vi "SetIMAvg.vi"(6 "Legacy (f)?":bool, 8 "error in (no error)":errorcluster, 10 "SetIMAvg":T1 items=["None", "Minimum", "Normal", "High", "Maximum"]) -> (0 "error out":errorcluster)   [LabVIEW 2011]
uses:
  HW Averaging.ctl
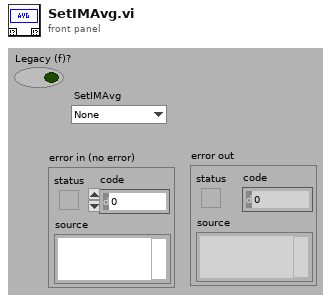
[diagram p1: front panel]
types:
  T1 = typedef "HW Averaging.ctl" = u16
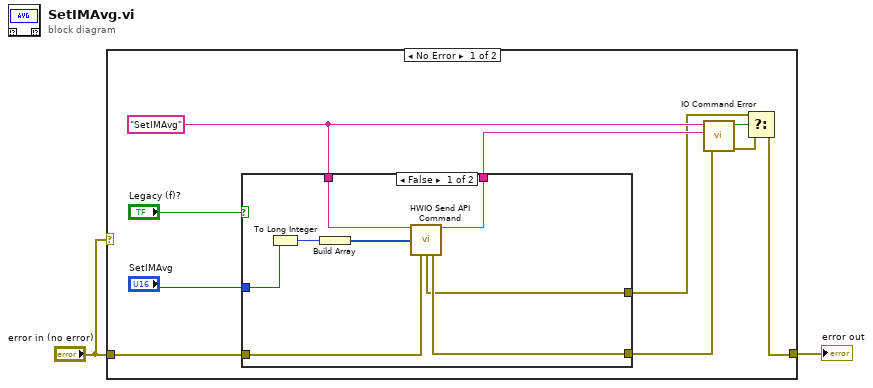
[diagram p0: block diagram]
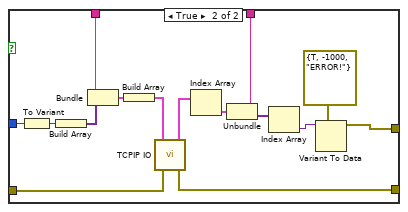
[diagram p2: hidden frame]
diagram:
  n1 = case shown="No Error" "error in (no error)" {
    tunnel: "error in (no error)" -> [w11 w36]
    tunnel: [w6 w36] -> w2
    frame No Error {
      w9 = "SetIMAvg"
      n2 = case shown="False" "Legacy (f)?" {
        tunnel: "SetIMAvg" -> [w16 w33]
        tunnel: w11 -> [w20 w32]
        tunnel: [w19 w30] -> w10
        tunnel: w9 -> [w17 w29]
        tunnel: [w18 w26] -> w8
        tunnel: [w13 w21] -> w4
        frame False {
          n3 = To Long Integer(number=w16) -> (32bit integer=w15:i32)
          n4 = Build Array(w15) -> (w14:i32[])
          n5 = call "HWIO Send API Command.vi"("Action"=w17, "Integer"=w14, "error in (no error)"=w20) -> ("Action out"=w18:string, "HWError"=w13:errorcluster, "error out"=w19:errorcluster)  [unwired: 5 in, 5 out]
        }
        frame True {
          n6 = To Variant(anything=w33) -> (Variant=w35:variant)
          n7 = Build Array(w35) -> (w34:variant[])
          n8 = Bundle(w29, w34) -> (w31:cluster{string, variant[]})  [unwired: 1 out]
          n9 = Build Array(w31) -> (w28:cluster{string, variant[]}[])
          n10 = call "TCPIP IO.vi"("error in (no error)"=w32, "Commands"=w28) -> ("error out"=w30:errorcluster, "Responses"=w25:cluster{string, variant[]}[])  [unwired: 1 in, 3 out]
          n11 = Index Array(array=w25) -> (element=w27:cluster{string, variant[]})  [unwired: 1 in]
          n12 = Unbundle(w27) -> (w26:string, w22:variant[])
          n13 = Index Array(array=w22) -> (element=w24:variant)  [unwired: 1 in]
          n14 = Variant To Data(type=errorcluster {"status"=TRUE, "code"=-1000, "source"="ERROR!"} ("error out"), Variant=w24) -> (data=w21:errorcluster)  [unwired: 1 in, 1 out]
        }
      }
      n15 = call "IO Command Error.vi"("error in (no error)"=w10, "Command Returned (\"\")"=w8, "Command Sent (\"\")"=w9) -> ("error out"=w5:errorcluster, "HW ERR?"=w7:bool)  [unwired: 3 out]
      n16 = Select(t=w4, s=w7, f=w5) -> (s? t:f=w6:errorcluster)
    }
    frame Error {
    }
  }
  "error out" <- w2
